vi "Monitor Flame.vi"(8 "error in":errorcluster, 9 "Flame Threshold":u32, 10 "Notifiers in":T1, 11 "Boiler Queue in":refnum<queue>) -> (0 "error out":errorcluster, 1 "Flame Level":u32, 2 "Notifiers out":T1, 3 "Boiler Queue out":refnum<queue>)   [LabVIEW 2022 SP3, in "Controller.lvlib"]
doc: "Monitor the flame level of the boiler until it is high enough to open the open the fuel control valve."
uses:
  Controller.lvlib
  Course Project/support/Message Queue/Message Cluster.ctl
  Course Project/support/Message Queue/Message Queue.lvlib
  support/Notifiers/Notifiers.ctl
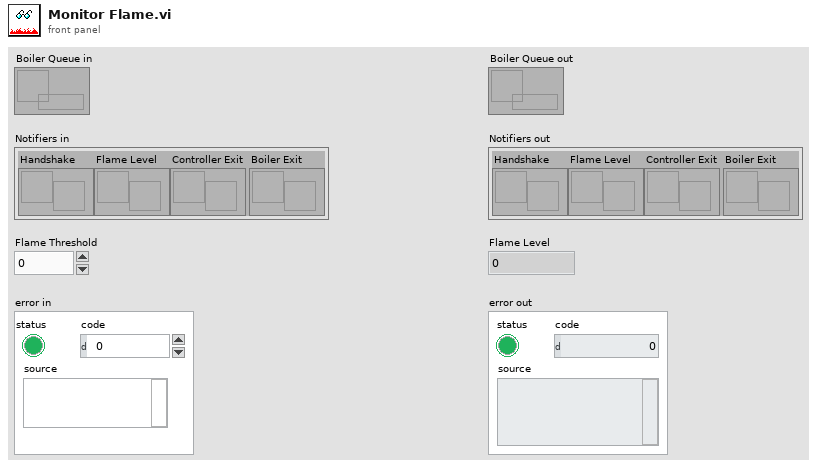
[diagram p1: front panel]
types:
  T1 = typedef "Notifiers.ctl" = cluster{"Handshake":refnum<notifier>, "Flame Level":refnum<notifier>, "Controller Exit":refnum<notifier>, "Boiler Exit":refnum<notifier>}
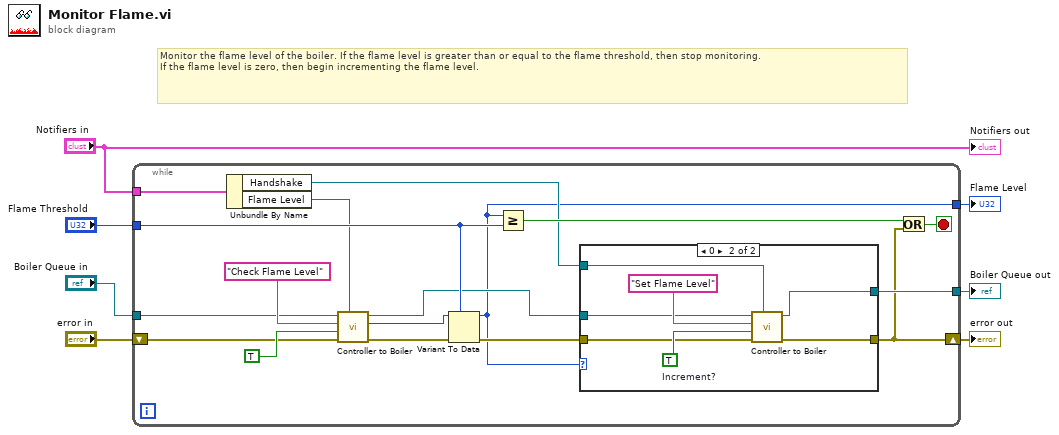
[diagram p0: block diagram]
diagram:
  # "Monitor the flame level of the boiler. If the flame level is greater than or equal to the flame threshold, then stop monitoring.\nIf the flame level is zero, then begin incrementing the flame level."
  n1 = while {
    tunnel: "Flame Threshold" -> [w24]
    tunnel: "Boiler Queue in" -> [w18]
    tunnel: [w8] -> w7
    shift-right: [w9] -> w1
    shift-left: "error in" -> [w19]
    tunnel: "Notifiers in" -> [w13]
    tunnel: [w10] -> w2
    stop <- w15 stop-if-true
    n2 = Unbundle By Name(w13) -> ("Handshake"=w11:refnum<notifier>, "Flame Level"=w12:refnum<notifier>)
    n3 = call "Controller to Boiler.vi"("Notifier"=w12, "error in"=w19, "Message Data"=TRUE, "Message"="Check Flame Level", "Boiler Queue in"=w18) -> ("error out"=w23:errorcluster, "notification"=w20:variant, "Queue out"=w16:refnum<queue>)  [unwired: 4 in]
    n4 = Variant To Data(error in=w23, type=w24, Variant=w20) -> (data=w8:u32, error out=w17:errorcluster)
    n5 = Greater Or Equal?(x=w8, y=w24) -> (x >= y?=w14:bool)
    n6 = case shown="0" w8 {
      tunnel: w17 -> [w26 w31]
      tunnel: [w26 w30] -> w9
      tunnel: w16 -> [w25 w29]
      tunnel: w11 -> [_ w28]
      tunnel: [w25 w27] -> w10
      frame Default {
      }
      frame 0 {
        w32 = TRUE  # Increment?
        n7 = call "Controller to Boiler.vi"("Notifier"=w28, "error in"=w31, "Message Data"=w32, "Message"="Set Flame Level", "Boiler Queue in"=w29) -> ("error out"=w30:errorcluster, "Queue out"=w27:refnum<queue>)  [unwired: 4 in, 1 out]
      }
    }
    n8 = Or(x=w14, y=w9) -> (x .or. y?=w15:bool)
  }
  "Flame Level" <- w7
  "Boiler Queue out" <- w2
  "error out" <- w1
  "Notifiers out" <- "Notifiers in"
